vi "Get and Set ToolsBar Property.vi"(8 "错误输入（无错误）":errorcluster, 9 "Mode":enum16{"Read", "Write"}(ring), 10 "ToolsBar In":T1, 11 "VI Ref In":refnum<vi>) -> (0 "错误输出":errorcluster, 2 "ToolsBar Out":T1, 3 "VI Ref Out":refnum<vi>)   [LabVIEW 2012, in "VIRef.lvlib"]
uses:
  VIRef.lvlib
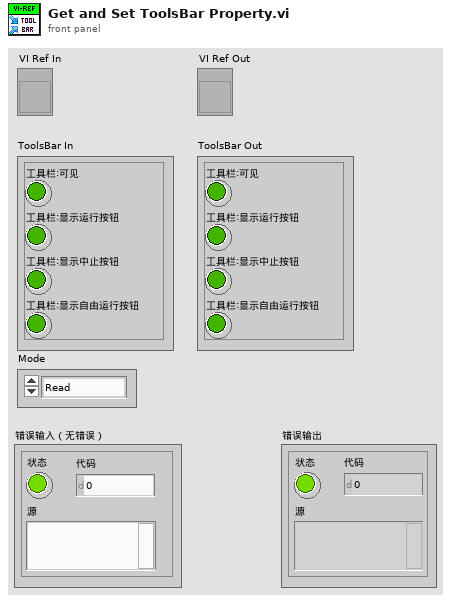
[diagram p1: front panel]
types:
  T1 = cluster{"工具栏:可见":bool, "工具栏:显示运行按钮":bool, "工具栏:显示中止按钮":bool, "工具栏:显示自由运行按钮":bool}
  T2 = cluster{"TB.Visible":bool, "TB.ShowRunBut":bool, "TB.ShowAbortBut":bool, "TB.ShowFreeRunBut":bool}
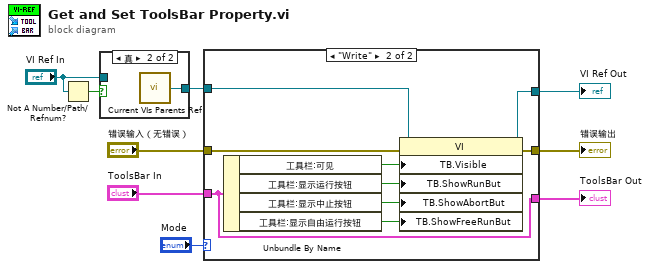
[diagram p0: block diagram]
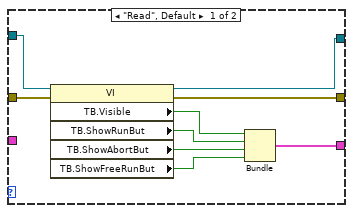
[diagram p2: hidden frame]
diagram:
  n1 = Not A Number/Path/Refnum?(number/path/refnum="VI Ref In") -> (NaN/Path/Refnum?=w8:bool)
  n2 = case shown="真" w8 {
    tunnel: [w10 w11] -> w4
    tunnel: "VI Ref In" -> [w10 _]
    frame False {
    }
    frame True {
      n3 = call "Current VIs Parents Ref.vi"() -> ("Calling VI's Reference"=w11:refnum<vi>)  [unwired: 2 in]
    }
  }
  n4 = case shown="\"Write\"" "Mode" {
    tunnel: "错误输入（无错误）" -> [w20 w28]
    tunnel: [w19 w26] -> w5
    tunnel: w4 -> [w18 w29]
    tunnel: [w17 w27] -> w3
    tunnel: "ToolsBar In" -> [_ w25]
    tunnel: [w12 w25] -> w1
    frame "Read", Default {
      n5 = property class="VI"(reference=w18, error in=w20) -> (reference out=w17:refnum<vi>, error out=w19:errorcluster, "TB.Visible"=w16:bool, "TB.ShowRunBut"=w15:bool, "TB.ShowAbortBut"=w14:bool, "TB.ShowFreeRunBut"=w13:bool)
      n6 = Bundle("TB.Visible"=w16, "TB.ShowRunBut"=w15, "TB.ShowAbortBut"=w14, "TB.ShowFreeRunBut"=w13) -> (w12:T2)  [unwired: 1 in]
    }
    frame "Write" {
      n7 = Unbundle By Name(w25) -> ("工具栏:可见"=w24:bool, "工具栏:显示运行按钮"=w23:bool, "工具栏:显示中止按钮"=w22:bool, "工具栏:显示自由运行按钮"=w21:bool)
      n8 = property class="VI"(reference=w29, error in=w28, "TB.Visible"=w24, "TB.ShowRunBut"=w23, "TB.ShowAbortBut"=w22, "TB.ShowFreeRunBut"=w21) -> (reference out=w27:refnum<vi>, error out=w26:errorcluster)
    }
  }
  "错误输出" <- w5
  "VI Ref Out" <- w3
  "ToolsBar Out" <- w1
